vi "Evaluate_version.vi"(8 "error in (no error)":errorcluster, 10 "min.expected":u64, 11 "Refnum in":T1) -> (0 "error out":errorcluster, 2 "dbg.lic.error":bool, 3 "Refnum out":T1)   [LabVIEW 2015, in "7976R_v1.lvclass"]
uses:
  <userlib>/SE-APP-Receiver/NI5772/7976R_v1/7976R_v1.lvclass
  <userlib>/SE-APP-Receiver/NI5772/7976R_v1/Private/FPGA VI Reference_DDC_v1.8.ctl
  <vilib>/Utility/error.llb/Error Cluster From Error Code.vi
  <vilib>/rvi/errors/niLvFpgaAdjustHostInterfaceError.vi
  <vilib>/rvi/interface/nirviReadWriteControl/nirviReadWriteControl.xnode
  <vilib>/rvi/interface/Simulation/niFpgaSimulationCallBeginRW.vi
  NiFpgaLv.dll
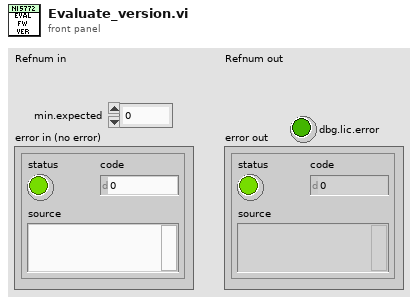
[diagram p1: front panel]
types:
  T1 = typedef "7976R_v1.lvclass/FPGA VI Reference_DDC_v1.8.ctl" = refnum<k20>
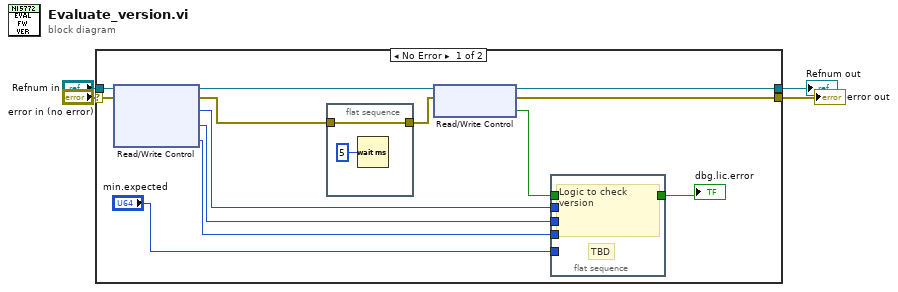
[diagram p0: block diagram]
diagram:
  n1 = case shown="No Error" "error in (no error)" {
    selector: "error in (no error)" -> [w16 w21]
    tunnel: "Refnum in" -> [w17 w22]
    tunnel: [w14 w22] -> w2
    tunnel: [w13 w21] -> w3
    frame No Error {
      n2 = xnode "Read/Write Control"("FPGA VI Reference In"=w17, "error in"=w16) -> ("FPGA VI Reference Out"=w15:T1, "error out"=w12:errorcluster, "ver.editorial"=w10:u8, "ver.technical"=w9:u8, "ver.major"=w8:u8)
      n3 = flat-sequence {
        tunnel: w12 -> [w19]
        tunnel: [w19] -> w11
        frame #0 {
          n4 = Wait (ms)(milliseconds to wait=u32 5) -> ()  [unwired: 1 out]
        }
      }
      n5 = xnode "Read/Write Control"("FPGA VI Reference In"=w15, "error in"=w11) -> ("FPGA VI Reference Out"=w14:T1, "error out"=w13:errorcluster, "dbg.lic.error"=w6:bool)
      n6 = flat-sequence {
        tunnel: w10 -> [_]
        tunnel: w9 -> [_]
        tunnel: w8 -> [_]
        tunnel: "min.expected" -> [_]
        tunnel: w6 -> [w18]
        tunnel: [w18] -> w5
        frame #0 {
          # "TBD"
          # "Logic to check version"
        }
      }
      "dbg.lic.error" <- w5
    }
    frame Error {
    }
  }
  "error out" <- w3
  "Refnum out" <- w2
